vi "Generate Dummy Channel Correction Text.vi"() -> (0 "Tables":string[](array[string]), 1 "Tables filenames":string[](array[string]), 2 "Tables directories":string[](array[string]), 3 "Channel correction file":string="% type of the correction\ntype:: channel\n\n% correction name string\nname:: generated by QPSCONTROL\n\n% device/channel identification as it appears in the digitizer identification\n% note: leave empty or remove if this correction should be independent of the instrument/channel\nchannel identifier::\n\n\n% nominal gain correction of the channel\n#startsection:: nominal gain\n\n  % scalar real value\n  #startmatrix:: value\n    1.000000\n  #endmatrix:: value\n  #startmatrix:: uncertainty\n    0.000025\n  #endmatrix:: uncertainty\n\n#endsection:: nominal gain\n\n% gain transfer\n#startsection:: gain transfer\n\n  % scalar real value\n  #startmatrix:: value\n    csv\\tfer_gain_50k.csv\n  #endmatrix:: value\n\n  // --- List of parameters on which the correction values depends: ---\n \t// primary parameter (remove if not used):\n \t#startsection:: primary parameter\n              \n    // name of the HW parameter:\n    //  note: it must be exact name of the parameter that appears in measurement header\n    name:: sampling rate [Sa/s]\n                                    \n    // is this parameter interpolable?\n    //  note: set to 0 or remove if not interpolable\n    interpolable:: 0\n                    \n    // list of supported values of a primary parameter on which the correction depends:\n    //  eg.: range of the digitizer\n    #startmatrix:: value\n      50000\n    #endmatrix:: value\n                \n  #endsection:: primary parameter\n\n#endsection:: gain transfer\n\n% input admittance\n#startsection:: input admittance\n\n  % CSV table with the 1D dependence on frequency\n  #startmatrix:: value\n    csv\\Y_inp.csv\n  #endmatrix:: value\n  \n#endsection:: input admittance\n\n% SFDR value\n#startsection:: sfdr\n\n  % CSV table with the 1D dependence on frequency\n  #startmatrix:: value\n    csv\\SFDR.csv\n  #endmatrix:: value\n  \n#endsection:: sfdr")   [LabVIEW 2020]
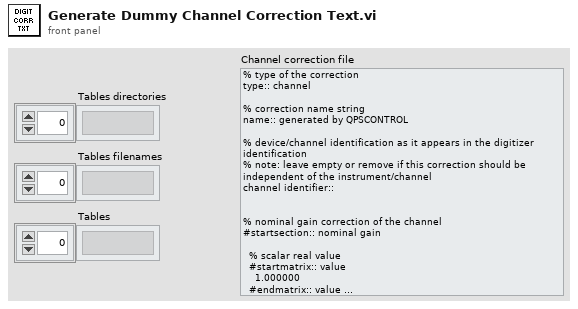
[diagram p1: front panel]
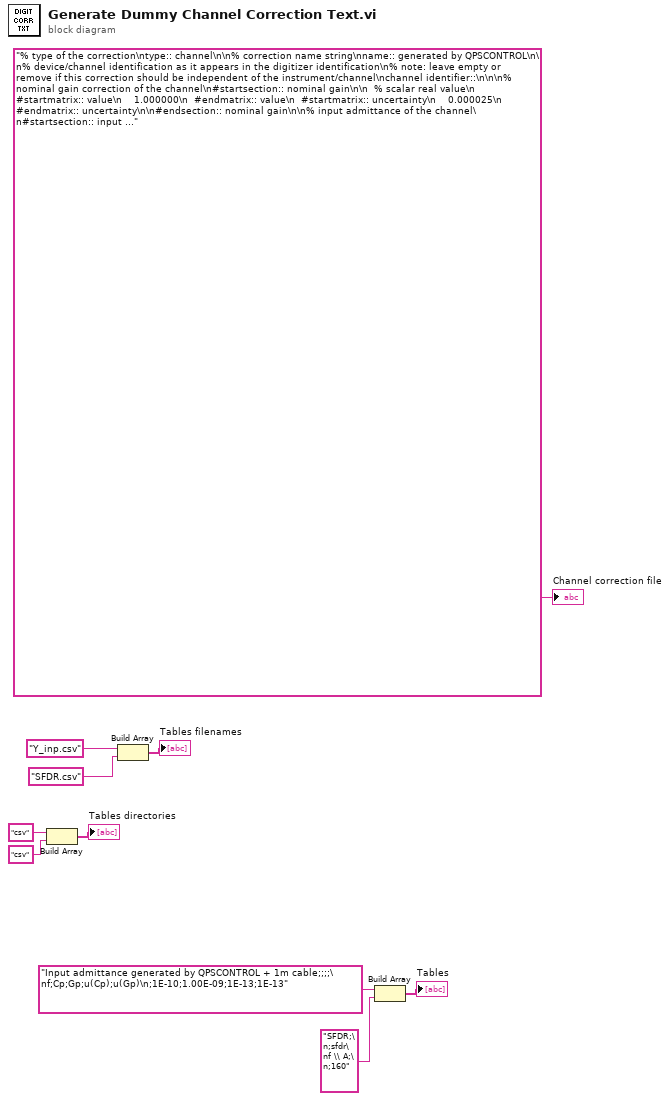
[diagram p0: block diagram]
diagram:
  n1 = Build Array("csv", "csv") -> (→"Tables directories":string[])
  n2 = Build Array("Y_inp.csv", "SFDR.csv") -> (→"Tables filenames":string[])
  n3 = Build Array("Input admittance generated by QPSCONTROL + 1m cable;;;;\nf;Cp;Gp;u(Cp);u(Gp)\n;1E-10;1.00E-09;1E-13;1E-13", "SFDR;\n;sfdr\nf \\ A;\n;160") -> (→"Tables":string[])
  "Channel correction file" <- "% type of the correction\ntype:: channel\n\n% correction name string\nname:: generated by QPSCONTROL\n\n% device/channel identification as it appears in the digitizer identification\n% note: leave empty or remove if this correction should be independent of the instrument/channel\nchannel identifier::\n\n\n% nominal gain correction of the channel\n#startsection:: nominal gain\n\n  % scalar real value\n  #startmatrix:: value\n    1.000000\n  #endmatrix:: value\n  #startmatrix:: uncertainty\n    0.000025\n  #endmatrix:: uncertainty\n\n#endsection:: nominal gain\n\n% input admittance of the channel\n#startsection:: input admittance\n\n  % CSV table with the 1D dependence on frequency\n  #startmatrix:: value\n    csv\\Y_inp.csv\n  #endmatrix:: value\n  \n#endsection:: input admittance\n\n% SFDR value\n#startsection:: sfdr\n\n  % CSV table with the 1D dependence on frequency\n  #startmatrix:: value\n    csv\\SFDR.csv\n  #endmatrix:: value\n  \n#endsection:: sfdr"
